vi "DeleteXMenuItem.vi"(8 "error in (no error)":errorcluster, 9 "ItemTag":string, 11 "CMenu in":refnum<class "CMenu.lvclass">) -> (0 "error out":errorcluster, 3 "CMenu out":refnum<class "CMenu.lvclass">)   [LabVIEW 2009]
doc: "Delete a Menu Item or SubMenu\n- ItemTag: Item which you want to deleted"
uses:
  CMenu.lvclass
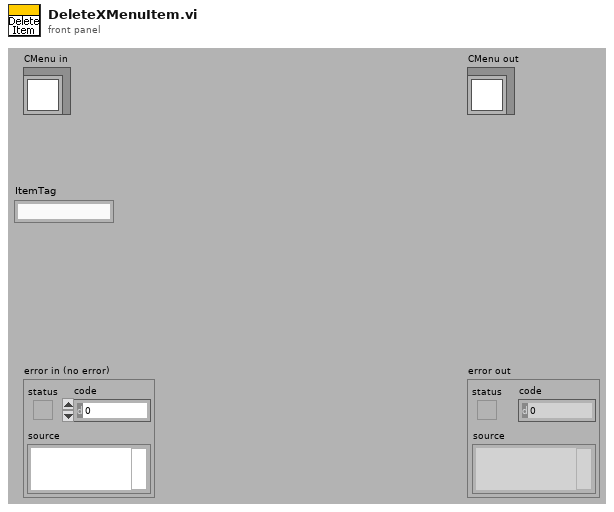
[diagram p1: front panel]
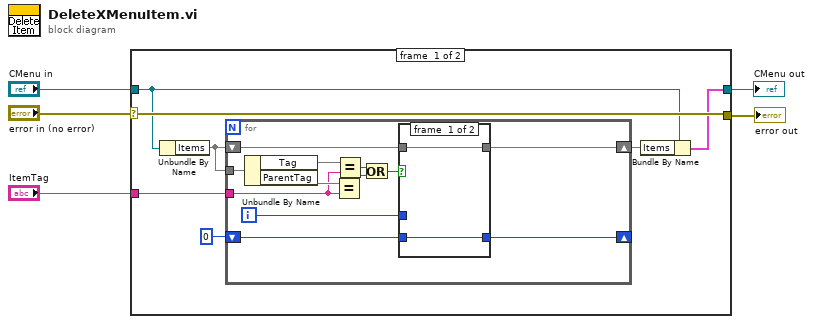
[diagram p0: block diagram]
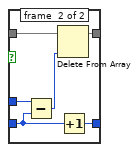
[diagram p2: hidden frame]
diagram:
  n1 = case shown="No Error" "error in (no error)" {
    selector: "error in (no error)" -> [w11 w34]
    tunnel: [w11 w34] -> w4
    tunnel: [w8 w33] -> w2
    tunnel: "CMenu in" -> [w9 w33]
    tunnel: "ItemTag" -> [w12 _]
    frame #0 {
      n2 = Unbundle By Name(w9) -> ("Items"=w6)
      n3 = for {
        tunnel: w12 -> [w22]
        shift-right: [w18] -> w10
        shift-left: w6 -> [w19]
        shift-right: [w15] -> _
        shift-left: 0 -> [w16]
        tunnel: w6 -> [w14]
        i -> [w13]
        n4 = Unbundle By Name(w14) -> ("Tag"=w24, "ParentTag"=w23)
        n5 = Equal?(x=w23, y=w22) -> (x = y?=w20:bool)
        n6 = Equal?(x=w24, y=w22) -> (x = y?=w21:bool)
        n7 = Or(x=w21, y=w20) -> (x .or. y?=w17:bool)
        n8 = case shown="True" w17 {
          tunnel: w19 -> [w26 w32]
          tunnel: [w26 w31] -> w18
          tunnel: w16 -> [w25 w29]
          tunnel: [w25 w30] -> w15
          tunnel: w13 -> [_ w28]
          frame #0 {
          }
          frame #1 {
            n9 = Subtract(x=w28, y=w29) -> (x-y=w27:i32)
            n10 = Delete From Array(array=w32, index=w27) -> (array with subset deleted=w31)  [unwired: 1 in, 1 out]
            n11 = Increment(x=w29) -> (x+1=w30:i32)
          }
        }
      }
      n12 = Bundle By Name(cluster=w9, "Items"=w10) -> (w8:cluster{})
    }
    frame #1 {
    }
  }
  "error out" <- w4
  "CMenu out" <- w2
